vi "qREL.vi"(0 "System no.":i32=1 min=1 max=4 step=1, 2 "Relays to query":string[](array[string]), 3 "All relays?":bool, 4 "Relay identifier?":bool=TRUE, 5 "error in":errorcluster) -> (14 "Relay status":bool[](array[boolean]), 19 "error out":errorcluster)   [LabVIEW 2020]
doc: "Returns relay status for queried relays.\n\nC-880: If All relays = TRUE, then Relay identifier can be FALSE."
panel:
  # "Returns relay status for queried relays."
  # "If all relays: use"
  # "Query"
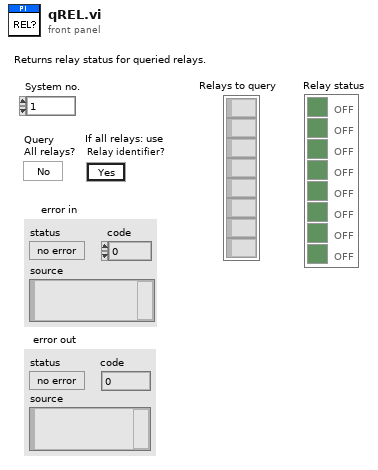
[diagram p1: front panel]
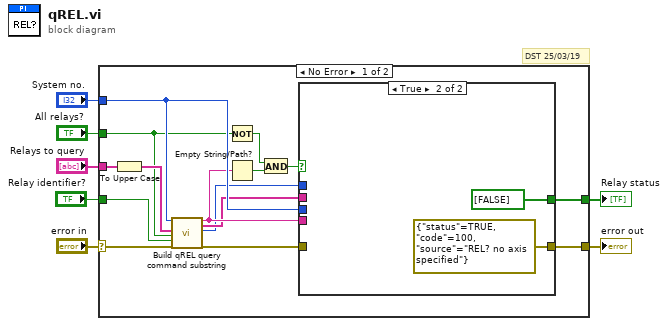
[diagram p0: block diagram]
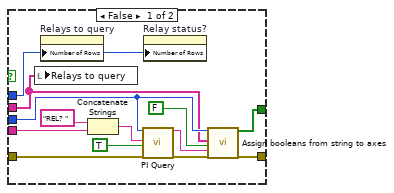
[diagram p2: hidden frame]
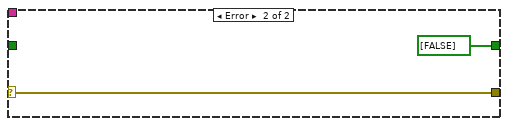
[diagram p3: hidden frame]
diagram:
  # "DST 25/03/19"
  n1 = case shown="No Error" "error in" {
    selector: "error in" -> [w10 w38]
    tunnel: [w22 bool[] [FALSE] ("Booleans")] -> w7
    tunnel: "Relays to query" -> [w21 _]
    tunnel: [w20 w38] -> w5
    tunnel: "Relay identifier?" -> [w18 _]
    tunnel: "System no." -> [w17 _]
    tunnel: "All relays?" -> [w14 _]
    frame No Error {
      n2 = To Upper Case(1:w21) -> (0:w19:string[])
      n3 = call "Build qREL query command substring.vi"("System no."=w17, "Relays to query in"=w19, "Query\nAll relays?"=w14, "For all relays: use\nRelay identifier?"=w18, "error in"=w10) -> ("Command substring"=w12:string, "Relays to query out"=w9:string[], "Number of rows"=w8:u32, "error out"=w15:errorcluster)  [unwired: 11 out]
      n4 = Not(x=w14) -> (.not. x?=w16:bool)
      n5 = Empty String/Path?(string/path=w12) -> (empty?=w11:bool)
      n6 = And(x=w16, y=w11) -> (x .and. y?=w13:bool)
      n7 = case shown="True" w13 {
        tunnel: [w32 bool[] [FALSE] ("Booleans")] -> w22
        tunnel: [w29 errorcluster {"status"=TRUE, "code"=100, "source"="REL? no axis specified"} ("error out")] -> w20
        tunnel: w12 -> [w31 _]
        tunnel: w17 -> [w30 _]
        tunnel: w9 -> [w23 _]
        tunnel: w15 -> [w28 _]
        tunnel: w8 -> [w24 _]
        frame False {
          n8 = local write "Relays to query"(w23) -> ()
          n9 = property on="Relays to query" class="Arr (strict)"("Number of Rows"=w24) -> ()  [unwired: 2 in, 2 out]
          n10 = Concatenate Strings("REL? ", w31) -> (w33:string)
          n11 = call "PI Query.vi"("System no."=w30, "String to send"=w33, "Attach termination char.?"=TRUE ("Attach Linefeed?"), "error in"=w28) -> ("String read"=w26:string, "error out"=w25:errorcluster)  [unwired: 3 in, 11 out]
          n12 = property on="Relay status?" class="Arr (strict)"("Number of Rows"=w24) -> ()  [unwired: 2 in, 2 out]
          n13 = call "Assign booleans from string to axes.vi"("System no."=w30, "Queried axes"=w23, "All axes queried?"=FALSE, "Input String"=w26, "error in"=w25) -> ("Booleans"=w32:bool[], "error out"=w29:errorcluster)  [unwired: 13 out]
        }
        frame True {
        }
      }
    }
    frame Error {
    }
  }
  "error out" <- w5
  "Relay status" <- w7
